vi "testVis.vi"() -> ()   [LabVIEW 2016]
panel:
  out "trimmed string":string
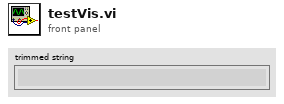
[diagram p1: front panel]
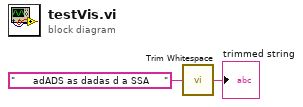
[diagram p0: block diagram]
diagram:
  n1 = call <vilib>:"Trim Whitespace.vi"("string"="      adADS as dadas d a SSA     ") -> ("trimmed string"=→"trimmed string":string)  [unwired: 1 in]
